vi "Example Simple.vi"() -> ()   [LabVIEW 2013]
uses:
  C:/tf/play/labview/Tinkerforge.dll
  Tinkerforge.dll
panel:
  out "uvi":sgl
  out "uvb (mW/m²)":sgl
  out "uva (mW/m²)":sgl
  in  "uid":string="amb"
  in  "port":i32=4223
  in  "host":string="localhost"
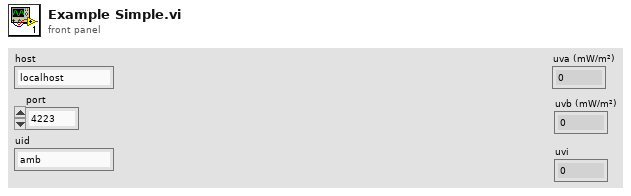
[diagram p1: front panel]
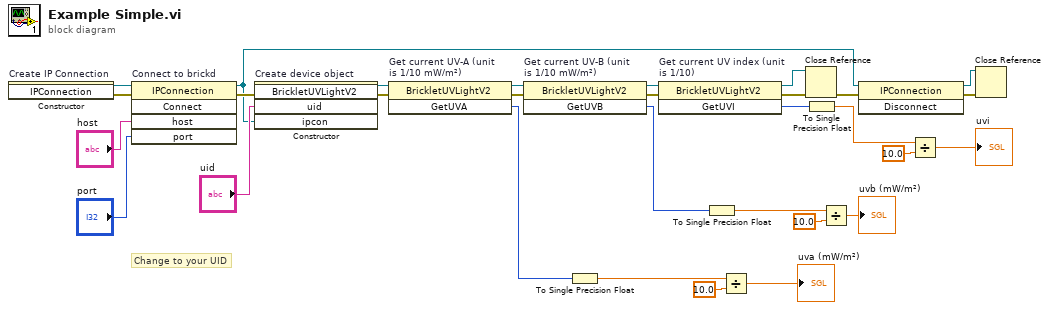
[diagram p0: block diagram]
diagram:
  # "Change to your UID"
  n1 = constructor on="Create IP Connection" class="IPConnection"() -> (reference out=w30:refnum<k24>, error out=w15:errorcluster)  [unwired: 3 in, 1 out]
  n2 = invoke on="Connect to brickd" class="IPConnection" method="Connect"(reference=w30, error in=w15, "host"="host", "port"="port") -> (reference out=w21:refnum<k24>, error out=w26:errorcluster)  [unwired: 1 in, 3 out]
  n3 = constructor on="Create device object" class="BrickletUVLightV2"(error in=w26, "uid"="uid", "ipcon"=w21) -> (reference out=w24:refnum<k24>, error out=w25:errorcluster)  [unwired: 2 in, 3 out]
  n4 = invoke on="Get current UV-A (unit\nis 1/10 mW/m²)" class="BrickletUVLightV2" method="GetUVA"(reference=w24, error in=w25) -> (reference out=w14:refnum<k24>, error out=w9:errorcluster, "GetUVA"=w19:i32)  [unwired: 1 in]
  n5 = invoke on="Get current UV-B (unit\nis 1/10 mW/m²)" class="BrickletUVLightV2" method="GetUVB"(reference=w14, error in=w9) -> (reference out=w13:refnum<k24>, error out=w10:errorcluster, "GetUVB"=w1:i32)  [unwired: 1 in]
  n6 = To Single Precision Float(number=w19) -> (single precision float=w17:sgl)
  n7 = invoke on="Get current UV index (unit\nis 1/10)" class="BrickletUVLightV2" method="GetUVI"(reference=w13, error in=w10) -> (reference out=w12:refnum<k24>, error out=w11:errorcluster, "GetUVI"=w2:i32)  [unwired: 1 in]
  n8 = To Single Precision Float(number=w1) -> (single precision float=w7:sgl)
  n9 = Divide(x=w17, y=sgl 10.0) -> (x/y=→"uva (mW/m²)":sgl)
  n10 = Close Reference(reference=w12, error in (no error)=w11) -> (error out=w23:errorcluster)
  n11 = To Single Precision Float(number=w2) -> (single precision float=w4:sgl)
  n12 = Divide(x=w7, y=sgl 10.0) -> (x/y=→"uvb (mW/m²)":sgl)
  n13 = invoke class="IPConnection" method="Disconnect"(reference=w21, error in=w23) -> (reference out=w20:refnum<k24>, error out=w22:errorcluster)  [unwired: 1 in, 1 out]
  n14 = Divide(x=w4, y=sgl 10.0) -> (x/y=→"uvi":sgl)
  n15 = Close Reference(reference=w20, error in (no error)=w22) -> ()  [unwired: 1 out]
